vi "Selected RT HW.vi"(8 "error in":errorcluster, 9 "Slctd HW IP":string[](array[string]), 10 "Slctd Hw Name":string[](array[string])) -> (0 "error out":errorcluster)   [LabVIEW 2018, in "Hardware Selection.lvlib"]
doc: "<b>Note</b>: This VI was renamed by the DQMH Rename Event utility. Make sure the VI Description is updated to reflect the new event name, then delete this comment.\n\nThis Broad cast event will send the Selected Hardware Detail's to other module's which regester's this module broadcast reference.\n_____\nCreated using DQMH Event Scripter 7.0.1.1316."
uses:
  Hardware Selection.lvlib
  Selected RT HW Argument--cluster.ctl
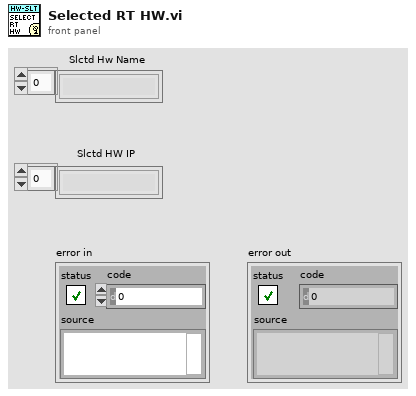
[diagram p1: front panel]
types:
  T1 = typedef "Hardware Selection.lvlib/Selected RT HW Argument--cluster.ctl" = cluster{"Slctd Hw Name":string[], "Slctd HW IP":string[]}
  T2 = typedef "Hardware Selection.lvlib/Broadcast Events--cluster.ctl" = cluster{"Module Did Init":refnum<user-event>, "Status Updated":refnum<user-event>, "Error Reported":refnum<user-event>, "Module Did Stop":refnum<user-event>, "Update Module Execution Status":refnum<user-event>, "Selected RT HW":refnum<user-event>}
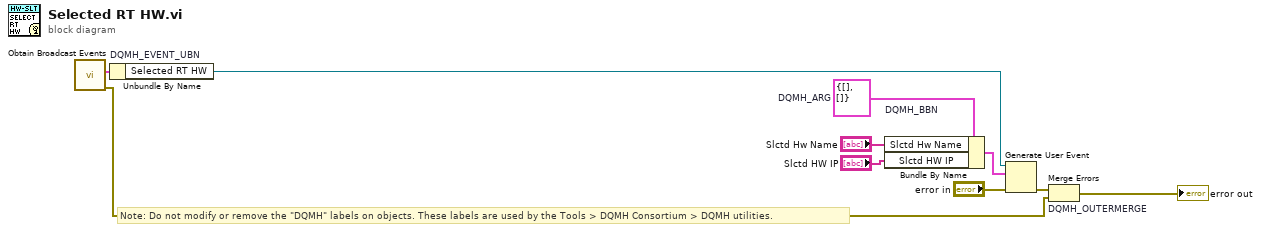
[diagram p0: block diagram]
diagram:
  w5 = T1 {"Slctd Hw Name"=[], "Slctd HW IP"=[]}  # DQMH_ARG
  # "Note: Do not modify or remove the \"DQMH\" labels on objects. These labels are used by the Tools > DQMH Consortium > DQMH utilities."
  n1 = call "Obtain Broadcast Events.vi"() -> ("error out"=w2:errorcluster, "Hardware Selection Broadcast Events"=w1:T2)  [unwired: 10 in]
  n2 = Unbundle By Name "DQMH_EVENT_UBN"(w1) -> ("Selected RT HW"=w7:refnum<user-event>)
  n3 = Bundle By Name "DQMH_BBN"(cluster=w5, "Slctd Hw Name"="Slctd Hw Name", "Slctd HW IP"="Slctd HW IP") -> (w8:T1)
  n4 = Generate User Event(user event=w7, event data cluster=w8, error in="error in") -> (error out=w6:errorcluster)  [unwired: 1 in, 1 out]
  n5 = Merge Errors "DQMH_OUTERMERGE"(w6, w2) -> (→"error out":errorcluster)
